vi "ProcessCommand.vi"(0 "MPUCommandFIFO":refnum<k21>, 1 "Command":u8, 2 "DebugFIFO":refnum<k21>, 3 "TelemetryFIFO":refnum<k21>, 4 "CommandsFIFO":refnum<k21>) -> ()   [LabVIEW 2018]
uses:
  <vilib>/rvi/DataTransferAndStorage/Container/Common/niFpgaContainerExecOnDevCompGetState.vi
  <vilib>/rvi/Emulation/niFpgaEmulationIsFPGAContextNoSignature.vi
  <vilib>/rvi/Emulation/niFpgaSctlEmulationGetInTimedLoop.vi
  <vilib>/rvi/errors/niFpgaSetErrorForExecOnDevCompSimple.vi
  <vilib>/rvi/eio/common/nirviEmuReportErrorAndStop.vi
  <vilib>/rvi/DataTransferAndStorage/Container/Common/niFpgaContainerGetUniqueNameForEmu.vi
  <vilib>/rvi/FIFO/Fifo_Resource/nirvififoEmulationSetSize.vi
  <vilib>/rvi/FIFO/Fifo_Resource/nirviFifoEmulationQueueMgr.vi
  <instcachedir>/0/nirviFifoEmulationQueueMgr_E5CAEC123FF24DC58D834DCA3CDAA9B5.lvgen/nirviFifoEmulationQueueMgr_E5CAEC123FF24DC58D834DCA3CDAA9B5_001.vi
  <vilib>/rvi/FIFO/Fifo_Resource/nirvififoEmulationDetermineInputValidOut.vi
  <vilib>/rvi/FIFO/Fifo_Resource/nirvififoEmulationCreateLock.vi
  <vilib>/rvi/Emulation/niFpgaProcessEmulError.vi
  <vilib>/rvi/FIFO/Fifo_Resource/nirvififoEmulationObtainLock.vi
  <vilib>/rvi/FIFO/Fifo_Resource/nirvififoEmulationReleaseLock.vi
  <vilib>/rvi/occurrence/nirviWaitOnOccurrenceBase.vi
  <vilib>/rvi/errors/nirviReportUnexpectedCaseInternalError.vi
  <vilib>/rvi/errors/nirviReportUnexpectedCaseInternalError (U32).vi
  <vilib>/Utility/error.llb/Clear Errors.vi
  <vilib>/rvi/interface/RandomDataEmulation/niFpgaRandomDataHandleErrors.vi
  <vilib>/rvi/Emulation/niFpgaGetClockAttributes.vi
  <vilib>/rvi/Emulation/niFpgaEmulationReportErrorSimple.vi
  <vilib>/rvi/Emulation/niFpgaCriticalErrorInLSC.vi
  <vilib>/rvi/DataTransferAndStorage/Container/XNode/niFpgaContainer.xnode
  <vilib>/rvi/FIFO/Fifo_Resource/niFpgaFifoEmulationRefIn.vi
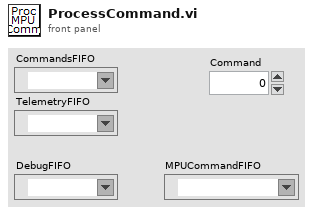
[diagram p1: front panel]
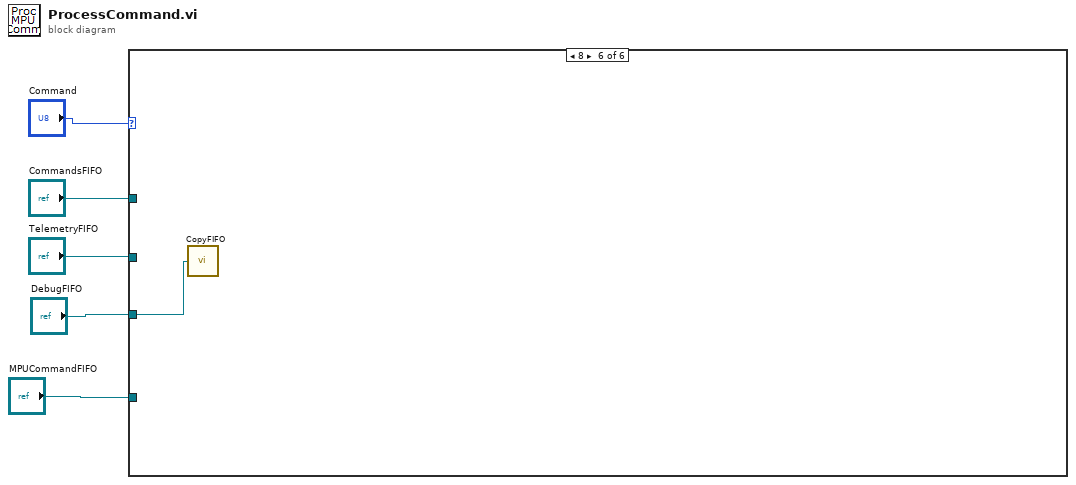
[diagram p0: block diagram]
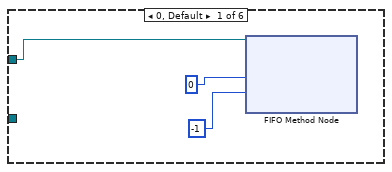
[diagram p2: hidden frame]
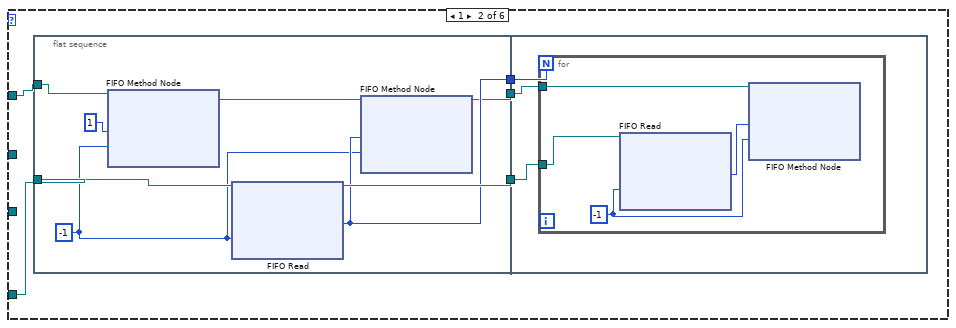
[diagram p3: hidden frame]
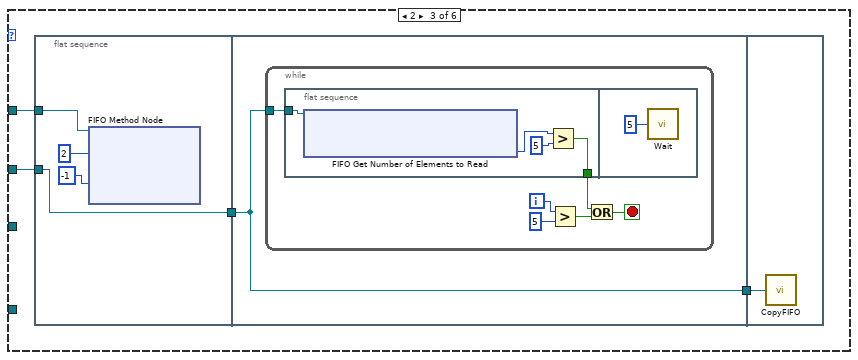
[diagram p4: hidden frame]
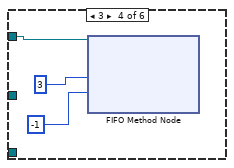
[diagram p5: hidden frame]
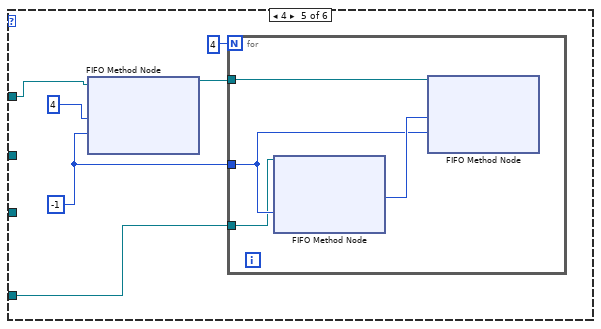
[diagram p6: hidden frame]
diagram:
  n1 = case shown="8" "Command" {
    tunnel: "MPUCommandFIFO" -> [_ w10 _ _ w54 _]
    tunnel: "CommandsFIFO" -> [w8 w9 w29 w50 w53 _]
    tunnel: "TelemetryFIFO" -> [_ _ w30 _ _ _]
    tunnel: "DebugFIFO" -> [_ _ _ _ _ w63]
    frame 0, Default {
      n2 = xnode ("FIFO Method Node")("Element"=0 ("Timeout"), "Timeout"=-1, "FIFO In"=w8) -> ()  [unwired: 2 out]
    }
    frame 1 {
      n3 = flat-sequence {
        tunnel: w10 -> [w21]
        tunnel: [w20] -> w13
        tunnel: [w19] -> w12
        tunnel: [w17] -> w11
        tunnel: w9 -> [w14]
        tunnel: w13 -> [w24]
        tunnel: w12 -> [w23]
        tunnel: w11 -> [w22]
        frame #0 {
          w15 = -1 ("Timeout")
          n4 = xnode ("FIFO Method Node")("Element"=u8 1, "Timeout"=w15, "FIFO In"=w14) -> ("FIFO Out"=w18:refnum<k21>)  [unwired: 1 out]
          n5 = xnode ("FIFO Read")("Timeout"=w15, "FIFO In"=w21) -> ("Element"=w19:u8, "FIFO Out"=w20:refnum<k21>)  [unwired: 1 out]
          n6 = xnode ("FIFO Method Node")("Element"=w19, "Timeout"=w15, "FIFO In"=w18) -> ("FIFO Out"=w17:refnum<k21>)  [unwired: 1 out]
        }
        frame #1 {
          n7 = for {
            N: w23 -> [_]
            tunnel: w24 -> [w26]
            tunnel: w22 -> [w25]
            w27 = -1 ("Timeout")
            n8 = xnode ("FIFO Read")("Timeout"=w27, "FIFO In"=w26) -> ("Element"=w28:u8)  [unwired: 2 out]
            n9 = xnode ("FIFO Method Node")("Element"=w28, "Timeout"=w27, "FIFO In"=w25) -> ()  [unwired: 2 out]
          }
        }
      }
    }
    frame 2 {
      n10 = flat-sequence {
        tunnel: [w34] -> w32
        tunnel: w30 -> [w34]
        tunnel: w29 -> [w33]
        tunnel: w32 -> [w37]
        tunnel: [w37] -> w31
        tunnel: w31 -> [w49]
        frame #0 {
          n11 = xnode ("FIFO Method Node")("Element"=2 ("Timeout"), "Timeout"=-1, "FIFO In"=w33) -> ()  [unwired: 2 out]
        }
        frame #1 {
          n12 = while {
            tunnel: w37 -> [w38]
            i -> [w41]
            stop <- w42 stop-if-true
            n13 = flat-sequence {
              tunnel: [w46] -> w43
              tunnel: w38 -> [w45]
              frame #0 {
                n14 = xnode ("FIFO Get Number of Elements to Read")("FIFO In"=w45) -> ("Number of Elements to Read"=w44:u32)  [unwired: 1 out]
                n15 = Greater?(x=w44, y=u32 5) -> (0:w46:bool)
              }
              frame #1 {
                n16 = call "Wait"("Count(mSec)"=u8 5) -> ()  [unwired: 1 out]
              }
            }
            n17 = Greater?(x=w41, y=5) -> (0:w39:bool)
            n18 = Or(x=w43, y=w39) -> (x .or. y?=w42:bool)
          }
        }
        frame #2 {
          n19 = call "CopyFIFO.vi"("Input"=w49) -> ()
        }
      }
    }
    frame 3 {
      n20 = xnode ("FIFO Method Node")("Element"=3 ("Timeout"), "Timeout"=-1, "FIFO In"=w50) -> ()  [unwired: 2 out]
    }
    frame 4 {
      w56 = -1 ("Timeout")
      n21 = xnode ("FIFO Method Node")("Element"=u8 4, "Timeout"=w56, "FIFO In"=w53) -> ("FIFO Out"=w55:refnum<k21>)  [unwired: 1 out]
      n22 = for {
        N: 4 -> [_]
        tunnel: w55 -> [w61]
        tunnel: w56 -> [w60]
        tunnel: w54 -> [w59]
        n23 = xnode ("FIFO Method Node")("Timeout"=w60, "FIFO In"=w59) -> ("Element"=w62:u8)  [unwired: 2 out]
        n24 = xnode ("FIFO Method Node")("Element"=w62, "Timeout"=w60, "FIFO In"=w61) -> ()  [unwired: 2 out]
      }
    }
    frame 8 {
      n25 = call "CopyFIFO.vi"("Input"=w63) -> ()
    }
  }
